vi "Create All Message Queues.vi"(8 "error in (no error)":errorcluster) -> (0 "error out":errorcluster, 3 "Message Queues out":T1)   [LabVIEW 2022 SP3, in "Message Queue.lvlib"]
doc: "This VI creates and initializes all the message queues for your application. If your application requires more than one message queue, right-click the \"Message Queues\" constant above and select Open Type Def. Add the new Message Queue(s) to the type definition, then initialize them in this VI."
uses:
  Message Queue.lvlib
  All Message Queues.ctl
  Message Cluster.ctl
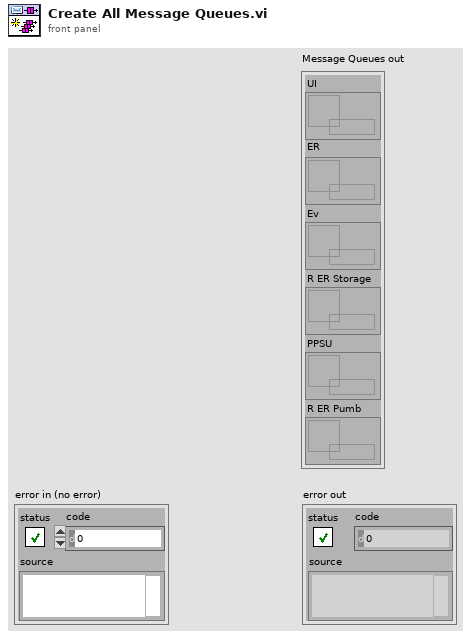
[diagram p1: front panel]
types:
  T1 = typedef "Message Queue.lvlib/All Message Queues.ctl" = cluster{"UI":refnum<queue>, "ER":refnum<queue>, "Ev":refnum<queue>, "R ER Storage":refnum<queue>, "PPSU":refnum<queue>, "R ER Pumb":refnum<queue>}
  T2 = cluster{"Error Code":string, "Error Source":string}
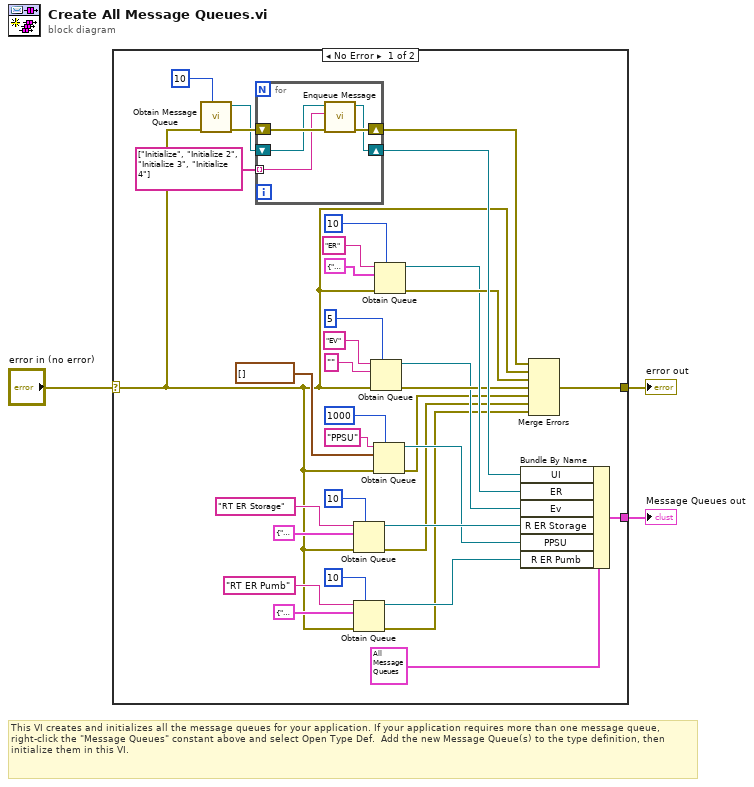
[diagram p0: block diagram]
diagram:
  # "This VI creates and initializes all the message queues for your application. If your application requires more than one message queue, right-click the \"Message Queues\" constant above and select Open Type Def.  Add the new Message Queue(s) to the type definition, then initialize them in this VI."
  n1 = case shown="No Error" "error in (no error)" {
    selector: "error in (no error)" -> [w4 w44]
    tunnel: [w32 w44] -> w3
    tunnel: [w36 _] -> w2
    frame No Error {
      n2 = call "Obtain Message Queue.vi"("max queue size (-1, unlimited)"=10, "error in (no error)"=w4) -> ("error out"=w35:errorcluster, "Message Queue"=w34:refnum<queue>)  [unwired: 8 in]
      n3 = for {
        tunnel: string[] ["Initialize", "Initialize 2", "Initialize 3", "Initialize 4"] ("Message") -> [w39] mode=indexing
        shift-right: [w43] -> w38
        shift-left: w35 -> [w42]
        shift-right: [w40] -> w33
        shift-left: w34 -> [w41]
        n4 = call "Enqueue Message.vi"("error in (no error)"=w42, "Message"=w39, "Message Queue"=w41) -> ("error out"=w43:errorcluster, "dup Message Queue"=w40:refnum<queue>)  [unwired: 7 in]
      }
      n5 = Obtain Queue(max queue size (-1, unlimited)=10, name (unnamed)="RT ER Storage", element data type=T2 {"Error Code"="", "Error Source"=""} ("element"), error in (no error)=w4) -> (queue out=w17:refnum<queue>, error out=w6:errorcluster)  [unwired: 1 in, 1 out]
      n6 = Obtain Queue(max queue size (-1, unlimited)=10, name (unnamed)="RT ER Pumb", element data type=T2 {"Error Code"="", "Error Source"=""} ("element"), error in (no error)=w4) -> (queue out=w7:refnum<queue>, error out=w5:errorcluster)  [unwired: 1 in, 1 out]
      n7 = Obtain Queue(max queue size (-1, unlimited)=5, name (unnamed)="EV", element data type="", error in (no error)=w4) -> (queue out=w18:refnum<queue>, error out=w23:errorcluster)  [unwired: 1 in, 1 out]
      n8 = Obtain Queue(max queue size (-1, unlimited)=1000, name (unnamed)="PPSU", element data type=waveform(dbl)[] [] ("Array"), error in (no error)=w4) -> (queue out=w12:refnum<queue>, error out=w11:errorcluster)  [unwired: 1 in, 1 out]
      n9 = Obtain Queue(max queue size (-1, unlimited)=10, name (unnamed)="ER", element data type=T2 {"Error Code"="", "Error Source"=""} ("element"), error in (no error)=w4) -> (queue out=w26:refnum<queue>, error out=w29:errorcluster)  [unwired: 1 in, 1 out]
      n10 = Bundle By Name(cluster=T1 {"UI"=refnum, "ER"=refnum, "Ev"=refnum, "R ER Storage"=refnum, "PPSU"=refnum, "R ER Pumb"=refnum} ("Message Queues"), "UI"=w33, "ER"=w26, "Ev"=w18, "R ER Storage"=w17, "PPSU"=w12, "R ER Pumb"=w7) -> (w36:T1)
      n11 = Merge Errors(w38, w4, w29, w23, w11, w6, w5) -> (w32:errorcluster)
    }
    frame Error {
    }
  }
  "Message Queues out" <- w2
  "error out" <- w3
